vi "SF2 Get Recording Status.vi"(7 "Update":bool, 11 "Recording (in)":bool) -> (3 "Recording (out)":bool)   [LabVIEW 2016]
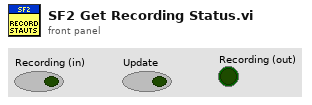
[diagram p1: front panel]
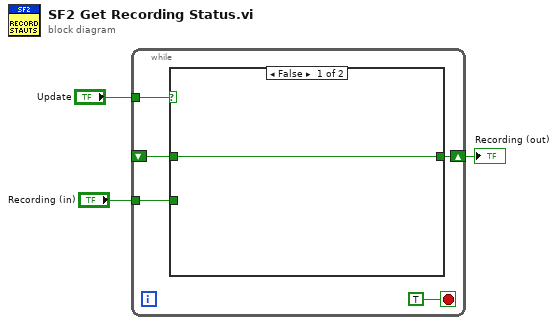
[diagram p0: block diagram]
diagram:
  n1 = while {
    tunnel: "Update" -> [w7]
    shift-right: [w5] -> w1
    shift-left: _ -> [w4]
    tunnel: "Recording (in)" -> [w6]
    stop <- TRUE stop-if-true
    n2 = case shown="False" w7 {
      tunnel: w6 -> [_ w10]
      tunnel: [w9 w10] -> w5
      tunnel: w4 -> [w9 _]
      frame False {
      }
      frame True {
      }
    }
  }
  "Recording (out)" <- w1
